vi "mb Convert [U8] to U32.vi"(2 "Data [ ]":u8[](array[numeric]), 4 "Byte Offset":u16=1) -> (6 "U32 Data [ ]":u32[](array[numeric]), 7 "U32 Data":u32)   [LabVIEW 2009]
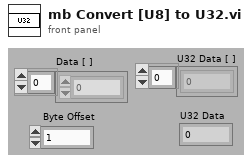
[diagram p1: front panel]
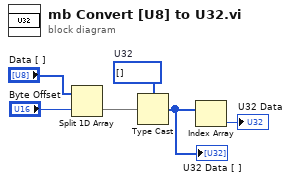
[diagram p0: block diagram]
diagram:
  w2 = u32[] []  # U32
  n1 = Split 1D Array(array="Data [ ]", index="Byte Offset") -> (second subarray=w3:u8[])  [unwired: 1 out]
  n2 = Type Cast(type=w2, x=w3) -> (*(type *) &x=w1:u32[])
  "U32 Data [ ]" <- w1
  n3 = Index Array(array=w1) -> (element=→"U32 Data":u32)  [unwired: 1 in]
